vi "ArmFieldLimit.vi"(9 "Extend Error":dbl, 10 "Lift Error":dbl, 11 "Going Down?":bool) -> (2 "Extend Error":dbl, 3 "Lift Error":dbl)   [LabVIEW 2020]
doc: "FIeld limit\nwhen going down ----\n when extend error is outside +/-1 then\n set lift error to 0\n (lift does not move)\nwhen going up ----\n when lift error is outside +/- 0.5 then\n set extend error to 0\n (extend doesn't move)"
uses:
  <vilib>/Rock Robotics/WPI/ThirdParty/JAS_Junk/TrajLib/Trajectory_Library.lvlib
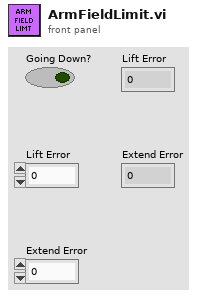
[diagram p1: front panel]
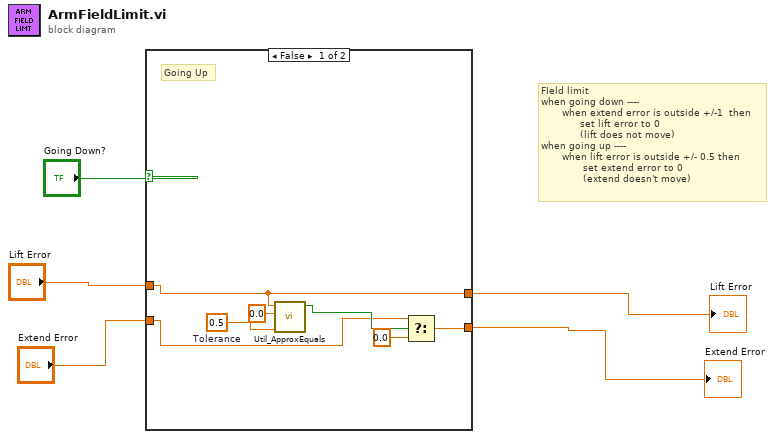
[diagram p0: block diagram]
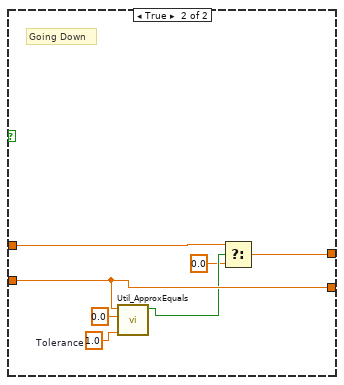
[diagram p2: hidden frame]
diagram:
  # "FIeld limit\nwhen going down ----\n       when extend error is outside +/-1  then\n             set lift error to 0\n             (lift does not move)\nwhen going up ----\n       when lift error is outside +/- 0.5 then\n              set extend error to 0\n              (extend doesn't move)"
  n1 = case shown="False" "Going Down?" {
    tunnel: "Extend Error" -> [w7 w18]
    tunnel: "Lift Error" -> [w9 w15]
    tunnel: [w12 w18] -> w4
    tunnel: [w9 w14] -> w5
    frame False {
      w10 = 0.5  # Tolerance
      # "Going Up"
      n2 = call <vilib>:"Util_ApproxEquals.vi"("Tolerance"=w10, "Value 2"=0.0, "Value 1"=w9) -> ("ApproxEquals"=w8:bool)  [unwired: 8 in]
      n3 = Select(t=w7, s=w8, f=0.0) -> (s? t:f=w12:dbl)
    }
    frame True {
      w17 = 1.0  # Tolerance
      # "Going Down"
      n4 = call <vilib>:"Util_ApproxEquals.vi"("Tolerance"=w17, "Value 2"=0.0, "Value 1"=w18) -> ("ApproxEquals"=w16:bool)  [unwired: 8 in]
      n5 = Select(t=w15, s=w16, f=0.0) -> (s? t:f=w14:dbl)
    }
  }
  "Lift Error" <- w5
  "Extend Error" <- w4
